vi "Close.vi"(8 "error in":errorcluster, 11 "Standard Engine in":refnum<class "Standard Engine Runtime.lvclass">) -> (0 "error out":errorcluster)   [LabVIEW 2013, in "Standard Engine Runtime.lvclass"]
uses:
  Standard Engine Runtime.lvclass
  <vilib>/NI/Module Execution Interface/Engine Runtime/Execution States.ctl
  Standard Engine Runtime.lvclass/Standard Engine Runtime.ctl
  Commands.ctl
  <vilib>/NI/Module Execution Interface/Engine Runtime/Engine Runtime Interface.lvclass
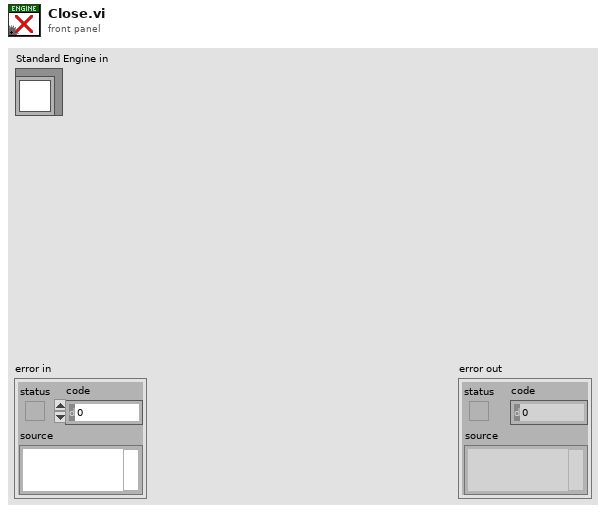
[diagram p1: front panel]
types:
  T1 = typedef "Engine Runtime Interface.lvclass/Execution States.ctl" = enum16{"Initializing", "Paused (Initialized)", "Running", "Set Safe Outputs", "Uninitializing", "Stopped (Uninitialized)", "Error (Uninitialized)", "Safe State (Uninitialized)", "Closed"}
  T2 = typedef "Standard Engine Runtime.lvclass/Engine VI Ref.ctl" = refnum<vi>
  T3 = typedef "Standard Engine Runtime.lvclass/Commands.ctl" = enum16{"Initialize", "Start", "Pause", "Safe State", "Normal", "Stop", "Shutdown"}
  T4 = enum32{"Bad", "Idle", "Run top level", "Running"}
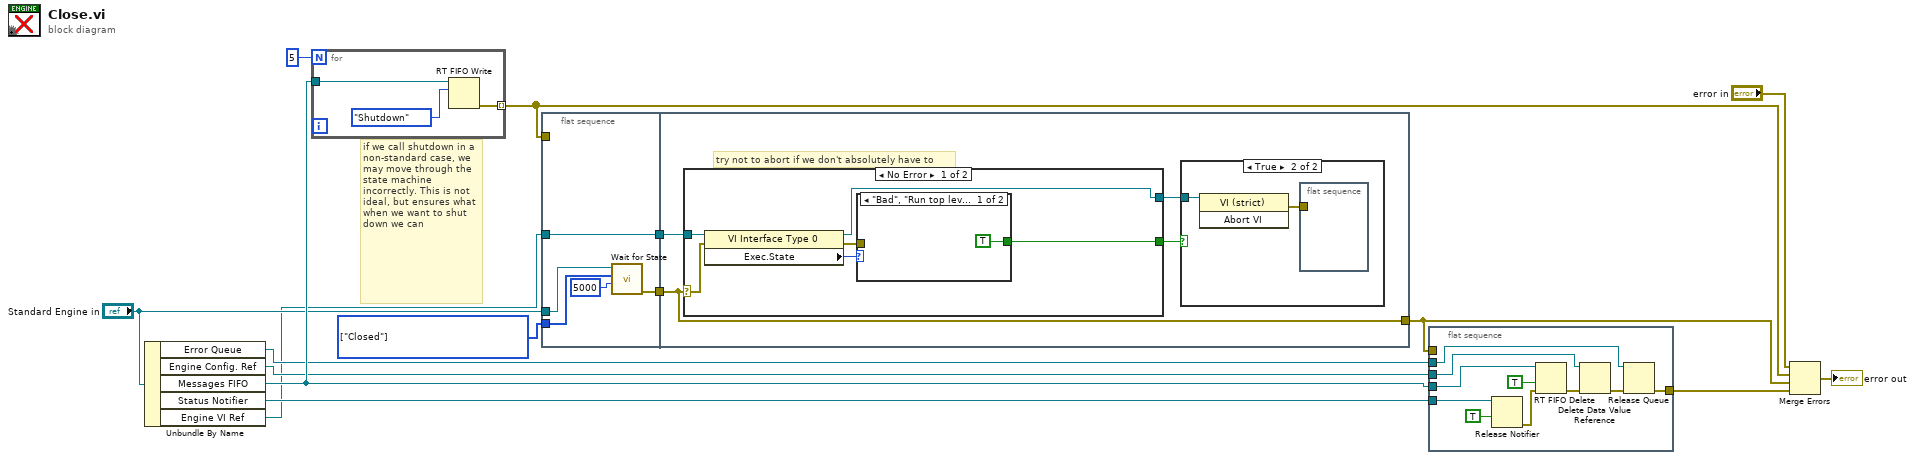
[diagram p0: block diagram]
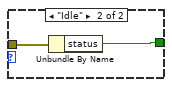
[diagram p3: hidden frame]
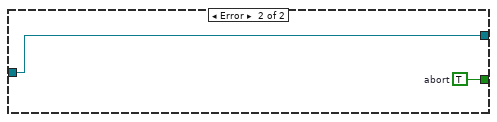
[diagram p4: hidden frame]
diagram:
  w13 = T1[] [enum."Closed"] items=["Initializing", "Paused (Initialized)", "Running", "Set Safe Outputs", "Uninitializing", "Stopped (Uninitialized)", "Error (Uninitialized)", "Safe State (Uninitialized)", "Closed"] ("expected states")
  # "if we call shutdown in a non-standard case, we may move through the state machine incorrectly. This is not ideal, but ensures what when we want to shut down we can"
  n1 = Unbundle By Name("Standard Engine in") -> ("Error Queue"=w7:refnum<queue>, "Engine Config. Ref"=w14:refnum<data-value>, "Messages FIFO"=w15:refnum<k33>, "Status Notifier"=w12:refnum<notifier>, "Engine VI Ref"=w3:T2)
  n2 = for {
    N: 5 -> [_]
    tunnel: w15 -> [w16]
    tunnel: [w17] -> w5 mode=indexing
    n3 = RT FIFO Write(0:w16, 1:Commands."Shutdown" ("element")) -> (11:w17:errorcluster)  [unwired: 3 in, 3 out]
  }
  n4 = flat-sequence {
    tunnel: w13 -> [w22]
    tunnel: "Standard Engine in" -> [w21]
    tunnel: w5 -> [_]
    tunnel: [w20] -> w4
    tunnel: w3 -> [w20]
    tunnel: [w19] -> w2
    tunnel: w4 -> [w26]
    tunnel: w2 -> [w27]
    tunnel: [w27] -> w1
    frame #0 {
      n5 = call "Wait for State.vi"("timeout in ms"=5000, "expected states"=w22, "Standard Engine in"=w21) -> ("error out"=w19:errorcluster)  [unwired: 7 in, 1 out]
    }
    frame #1 {
      # "try not to abort if we don't absolutely have to"
      n6 = case shown="No Error" w27 {
        selector: w27 -> [w34 _]
        tunnel: [w31 w40] -> w25
        tunnel: w26 -> [w35 w39]
        tunnel: [w30 w39] -> w24
        frame No Error {
          n7 = property class="VI Interface Type 0"(reference=w35, error in=w34) -> (reference out=w30:T2, error out=w32:errorcluster, "Exec.State"=w33:T4)
          n8 = case shown="\"Bad\", \"Run top level\", \"Running\"" w33 {
            tunnel: w32 -> [_ w38]
            tunnel: [TRUE ("status") w37] -> w31
            frame "Bad", "Run top level", "Running" {
            }
            frame "Idle" {
              n9 = Unbundle By Name(w38) -> ("status"=w37:bool)
            }
          }
        }
        frame Error {
          w40 = TRUE  # abort
        }
      }
      n10 = case shown="True" w25 {
        tunnel: w24 -> [_ w29]
        frame False {
        }
        frame True {
          n11 = invoke class="VI (strict)" method="Abort VI"(reference=w29) -> (error out=w28:errorcluster)  [unwired: 2 in, 2 out]
          n12 = flat-sequence {
            tunnel: w28 -> [_]
            frame #0 {
            }
          }
        }
      }
    }
  }
  n13 = flat-sequence {
    tunnel: w15 -> [w50]
    tunnel: w14 -> [w47]
    tunnel: w12 -> [w45]
    tunnel: [w42] -> w8
    tunnel: w7 -> [w41]
    tunnel: w1 -> [_]
    frame #0 {
      n14 = Release Notifier(notifier=w45, force destroy? (F)=TRUE) -> (error out=w44:errorcluster)  [unwired: 1 in, 2 out]
      n15 = RT FIFO Delete(0:w50, 2:TRUE ("force destroy? (F)"), 3:w44) -> (11:w49:errorcluster)
      n16 = Delete Data Value Reference(data value reference=w47, error in=w49) -> (error out=w43:errorcluster)  [unwired: 1 out]
      n17 = Release Queue(queue=w41, error in (no error)=w43) -> (error out=w42:errorcluster)  [unwired: 1 in, 2 out]
    }
  }
  n18 = Merge Errors("error in", w5, w1, w8) -> (→"error out":errorcluster)
